vi "写入全部.vi"(0 "表格控件":string[][](table)) -> ()   [LabVIEW 2016]
doc: "本VI通过将表格写入Excel工作表说明利用OLE自动化VI的基本方式。"
panel:
  in  "Completion Task":u16(ring) caption="完成任务" items=["保持Excel打开", "关闭电子表格"]
  out "error out":errorcluster caption="错误输出"
  in  "error in (no error)":errorcluster caption="错误输入（无错误）"
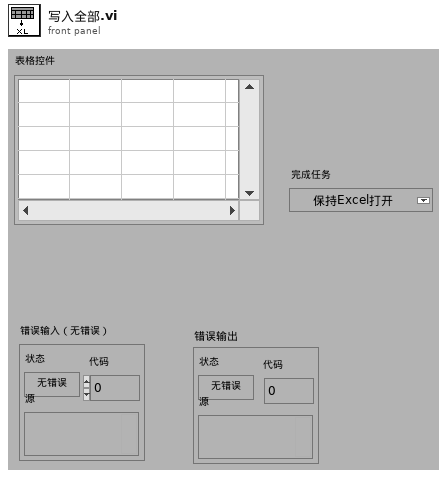
[diagram p1: front panel]
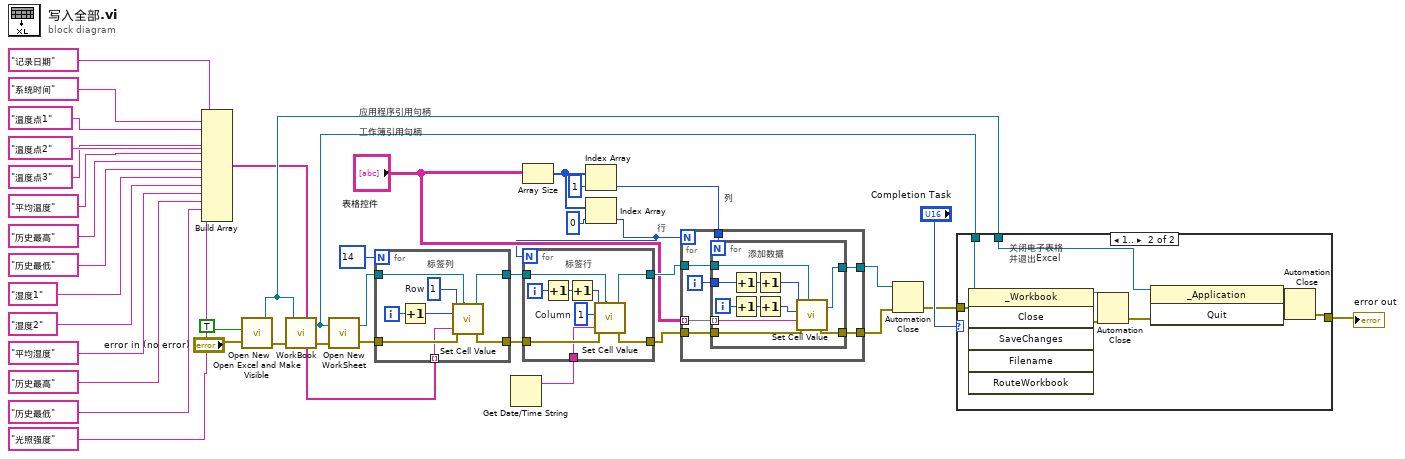
[diagram p0: block diagram]
diagram:
  # "列"
  # "行"
  # "工作簿引用句柄"
  # "应用程序引用句柄"
  n1 = Build Array("记录日期", "系统时间", "温度点1", "温度点2", "温度点3", "平均温度", "历史最高", "历史最低", "湿度1", "湿度2", "平均湿度", "历史最高", "历史最低", "光照强度") -> (w21:string[])
  n2 = call "Open Excel and Make Visible.vi"("error in (no error)"="error in (no error)", "Visible Boolean"=TRUE) -> ("error out"=w35:errorcluster, "Excel._Application"=w30:refnum<k7>)
  n3 = call "Open New  WorkBook.vi"("error in (no error)"=w35, "Excel._Application"=w30) -> ("error out"=w34:errorcluster, "Excel._Workbook"=w31:refnum<k7>)  [unwired: 1 out]
  n4 = call "Open New WorkSheet.vi"("error in (no error)"=w34, "Excel._Workbook"=w31) -> ("error out"=w25:errorcluster, "Excel._Worksheet"=w26:refnum<k7>)  [unwired: 1 out]
  n5 = for {
    N: 14 -> [_]
    tunnel: w26 -> [w47]
    tunnel: w25 -> [w46]
    tunnel: [w45] -> w19
    tunnel: [w44] -> w17
    tunnel: w21 -> [w42] mode=indexing
    i -> [w48]
    w43 = 1  # Row
    # "标签列"
    n6 = Increment(x=w48) -> (x+1=w41:i32)
    n7 = call "Set Cell Value.vi"("Row"=w43, "Col"=w41, "Value"=w42, "error in (no error)"=w46, "Excel._Worksheet"=w47) -> ("Excel._Worksheet"=w44:refnum<k7>, "error out"=w45:errorcluster)
  }
  n8 = Get Date/Time String() -> (date string=w15:string)  [unwired: 3 in, 1 out]
  n9 = Array Size(array="表格控件") -> (size(s)=w40:i32[])
  n10 = Index Array(array=w40, index=1) -> (element=w33:i32)
  n11 = Index Array(array=w40, index=0) -> (element=w10:i32)
  n12 = for {
    N: w10 -> [_]
    tunnel: w17 -> [w53]
    tunnel: w19 -> [w52]
    tunnel: [w51] -> w18
    tunnel: [w50] -> w16
    tunnel: w15 -> [w49]
    i -> [w57]
    w55 = 1  # Column
    # "标签行"
    n13 = Increment(x=w57) -> (x+1=w56:i32)
    n14 = Increment(x=w56) -> (x+1=w54:i32)
    n15 = call "Set Cell Value.vi"("Row"=w54, "Col"=w55, "Value"=w49, "error in (no error)"=w52, "Excel._Worksheet"=w53) -> ("Excel._Worksheet"=w50:refnum<k7>, "error out"=w51:errorcluster)
  }
  n16 = for {
    N: w10 -> [_]
    tunnel: w16 -> [w64]
    tunnel: w18 -> [w62]
    tunnel: [w63] -> w29
    tunnel: "表格控件" -> [w61] mode=indexing
    tunnel: w33 -> [w60]
    tunnel: [w59] -> w27
    i -> [w58]
    n17 = for {
      N: w60 -> [_]
      tunnel: w64 -> [w71]
      tunnel: w62 -> [w70]
      tunnel: [w69] -> w63
      tunnel: w58 -> [w68]
      tunnel: w61 -> [w67] mode=indexing
      tunnel: [w66] -> w59
      i -> [w75]
      # "添加数据"
      n18 = Increment(x=w68) -> (x+1=w74:i32)
      n19 = Increment(x=w75) -> (x+1=w72:i32)
      n20 = Increment(x=w74) -> (x+1=w73:i32)
      n21 = Increment(x=w72) -> (x+1=w65:i32)
      n22 = call "Set Cell Value.vi"("Row"=w73, "Col"=w65, "Value"=w67, "error in (no error)"=w70, "Excel._Worksheet"=w71) -> ("Excel._Worksheet"=w66:refnum<k7>, "error out"=w69:errorcluster)
    }
  }
  n23 = Automation Close(3:w29, 5:w27) -> (0:w28:errorcluster)
  n24 = case shown="1.." "Completion Task" {
    tunnel: [w76 w77] -> w11
    tunnel: w31 -> [_ w85]
    tunnel: w30 -> [_ w81]
    tunnel: w28 -> [w76 w84]
    frame ..0 {
    }
    frame 1.. {
      # "关闭电子表格\n并退出Excel"
      n25 = invoke class="_Workbook" method="Close"(reference=w85, error in=w84) -> (reference out=w83:refnum<k7>, error out=w82:errorcluster)  [unwired: 4 in, 4 out]
      n26 = Automation Close(3:w82, 5:w83) -> (0:w80:errorcluster)
      n27 = invoke class="_Application" method="Quit"(reference=w81, error in=w80) -> (reference out=w78:refnum<k7>, error out=w79:errorcluster)  [unwired: 1 in, 1 out]
      n28 = Automation Close(3:w79, 5:w78) -> (0:w77:errorcluster)
    }
  }
  "error out" <- w11
